vi "Main Page Name.vi"() -> (3 "name":string)   [LabVIEW 2019, in "DSF Shared.lvlib"]
uses:
  DSF Shared.lvlib
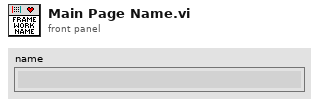
[diagram p1: front panel]
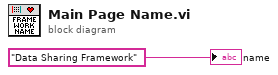
[diagram p0: block diagram]
diagram:
  "name" <- "Data Sharing Framework" ("Name")
